vi "Set Events.vi"(7 "Actor in":refnum<class "Actor.lvclass">, 11 "Dev Panel in":refnum<class "Dev Panel.lvclass">) -> (5 "Actor out":refnum<class "Actor.lvclass">)   [LabVIEW 2021, in "Dev Panel.lvclass"]
uses:
  Dev Panel.lvclass
  <vilib>/jettl/jettl/Actor/Actor/Actor.lvclass
  Dev Panel.lvclass/Dev Panel.ctl
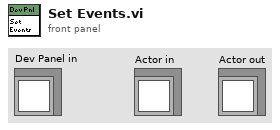
[diagram p1: front panel]
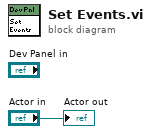
[diagram p0: block diagram]
diagram:
  "Actor out" <- "Actor in"
